vi "Init UART.vi"(4 "RX GPIO":u8=1, 5 "Term Char (None)":string, 6 "TX GPIO":u8, 7 "UART":u8, 8 "error in (no error)":errorcluster, 10 "Baud":u32=115200, 11 "VISA resource name in":refnum<visa-resource-name>) -> (0 "error out":errorcluster, 3 "VISA resource name":refnum<visa-resource-name>)   [LabVIEW 2024, in "CTIPicoVISA.lvlib"]
uses:
  CTIPicoVISA.lvlib
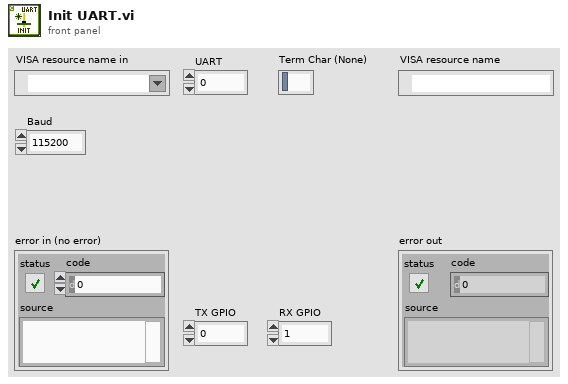
[diagram p1: front panel]
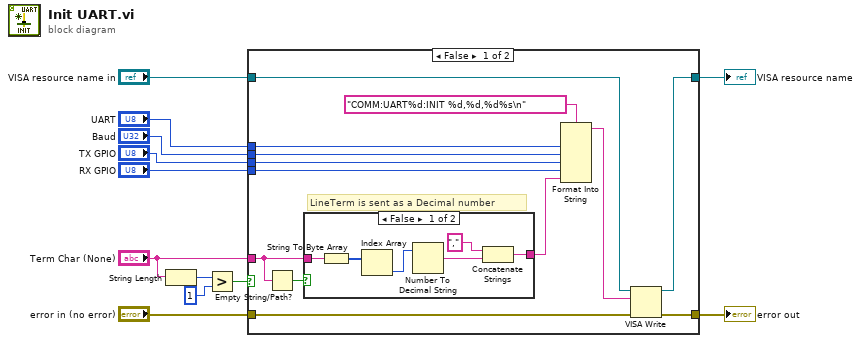
[diagram p0: block diagram]
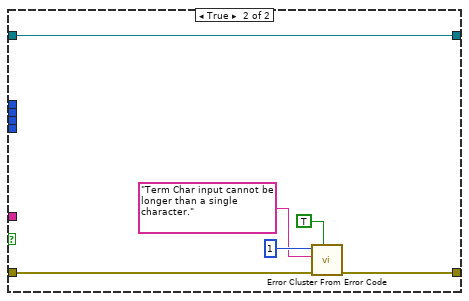
[diagram p3: hidden frame]
diagram:
  n1 = String Length(string="Term Char (None)") -> (length=w8:i32)
  n2 = Greater?(x=w8, y=1) -> (0:w6:bool)
  n3 = case shown="False" w6 {
    tunnel: "UART" -> [w24 _]
    tunnel: "Baud" -> [w23 _]
    tunnel: "TX GPIO" -> [w22 _]
    tunnel: "RX GPIO" -> [w21 _]
    tunnel: "Term Char (None)" -> [w19 _]
    tunnel: "error in (no error)" -> [w18 w36]
    tunnel: [w17 w35] -> w3
    tunnel: "VISA resource name in" -> [w16 w37]
    tunnel: [w15 w37] -> w1
    frame False {
      # "LineTerm is sent as a Decimal number"
      n4 = Empty String/Path?(string/path=w19) -> (empty?=w20:bool)
      n5 = case shown="False" w20 {
        tunnel: w19 -> [w29 _]
        tunnel: [w31 _] -> w14
        frame False {
          n6 = String To Byte Array(string=w29) -> (unsigned byte array=w28:u8[])
          n7 = Index Array(array=w28) -> (element=w27:u8)  [unwired: 1 in]
          n8 = Number To Decimal String(number=w27) -> (decimal integer string=w26:string)  [unwired: 1 in]
          n9 = Concatenate Strings("," ("string"), w26) -> (w31:string)
        }
        frame True {
        }
      }
      n10 = Format Into String(format string="COMM:UART%d:INIT %d,%d,%d%s\n", w24, w23, w22, w21, w14) -> (resulting string=w13:string)  [unwired: 2 in, 1 out]
      n11 = VISA Write(VISA resource name=w16, write buffer=w13, error in (no error)=w18) -> (VISA resource name out=w15:refnum<visa-resource-name>, error out=w17:errorcluster)  [unwired: 1 out]
    }
    frame True {
      n12 = call <vilib>:"Error Cluster From Error Code.vi"("show call chain? (False)"=TRUE, "error in (no error)"=w36, "error message (\"\")"="Term Char input cannot be longer than a single character.", "error code (0)"=1) -> ("error out"=w35:errorcluster)  [unwired: 5 in]
    }
  }
  "VISA resource name" <- w1
  "error out" <- w3
